vi "loadRecipeOthers.vi"() -> ()   [LabVIEW 2012]
uses:
  <vilib>/Utility/NIReport.llb/NI_report.lvclass
  <vilib>/addons/database/Connection.llb/DB Tools Open Connec (Path).vi
  <vilib>/addons/database/Connection.llb/Conn Execute.vi
  <vilib>/addons/database/Recordset.llb/Rec Destroy - Connection.vi
  <vilib>/Utility/NIReport.llb/Excel/NI_Excel.lvclass
  <vilib>/addons/database/NI_Database_API.lvlib
panel:
  in  "path":path=path "O:/Monitor/Recipe/OTHERS"
  out "filenames":string[](array[string])
  out "appended path":path
  out "data":string[][](array[string])
  out "error out 4":errorcluster
  in  "Cluster":T1
  out "error out 3":errorcluster
  in  "start cell":string="a2"
  out "error out":errorcluster
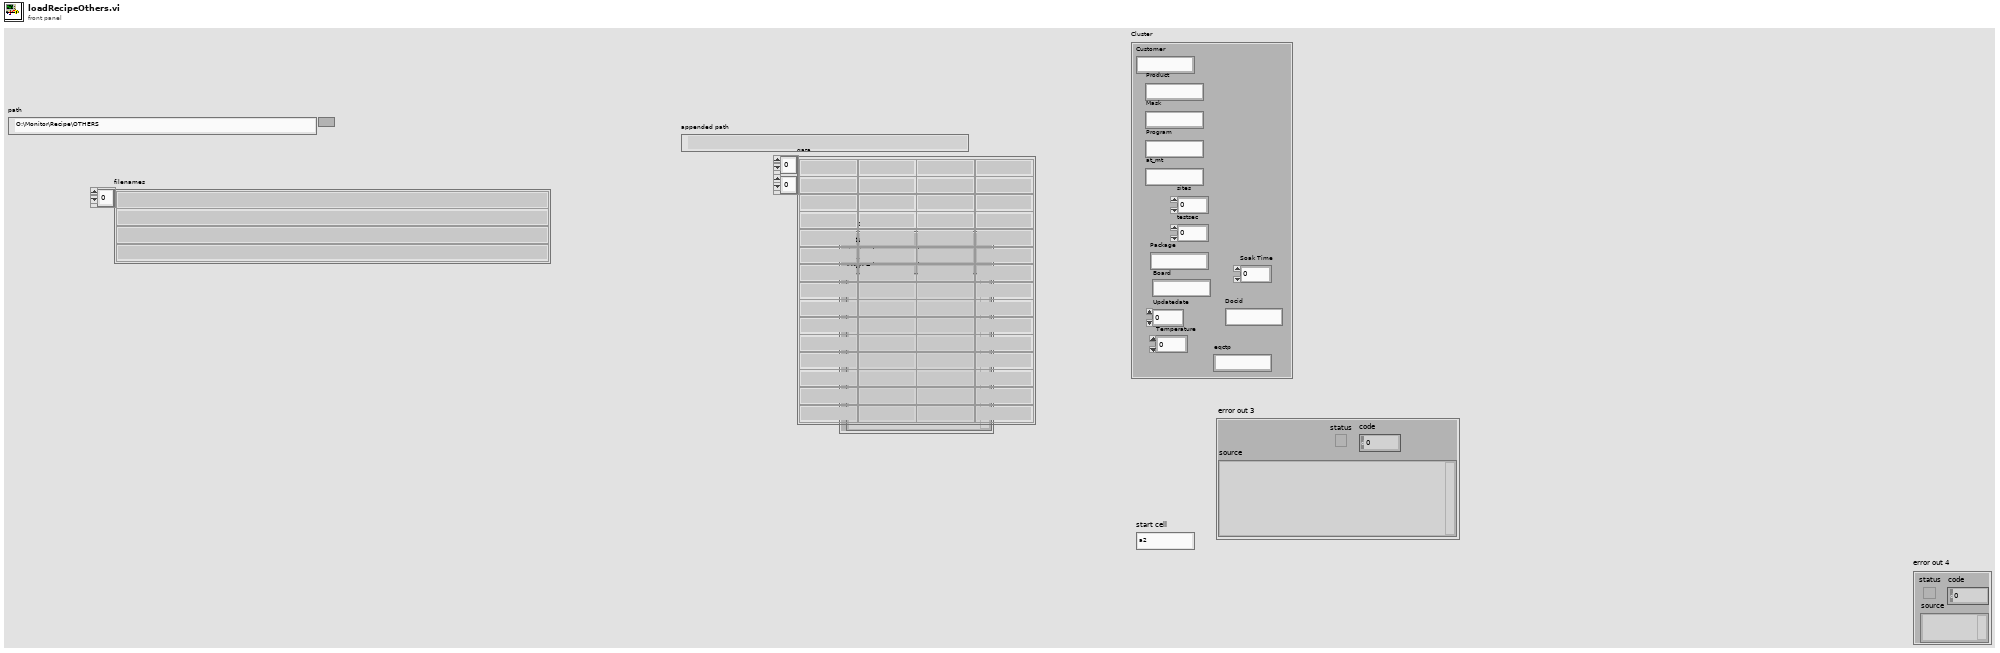
[diagram p1: front panel]
types:
  T1 = cluster{"Customer ":string, "Product":string, "Mask":string, "Program":string, "at_mt":string, "sites ":dbl, "testsec":dbl, "Package":string, "Board ":string, "Updatedate ":dbl, "Temperature":dbl, "Soak Time":dbl, "Docid":string, "eqctp":string}
  T2 = enum16{"Standard Report", "HTML", "Word", "Excel"}
  T3 = typedef "NI_Database_API.lvlib/Conn ObjectReference.ctl" = refnum<k1>
  T4 = typedef "NI_Database_API.lvlib/Rec ObjectReference.ctl" = refnum<k1>
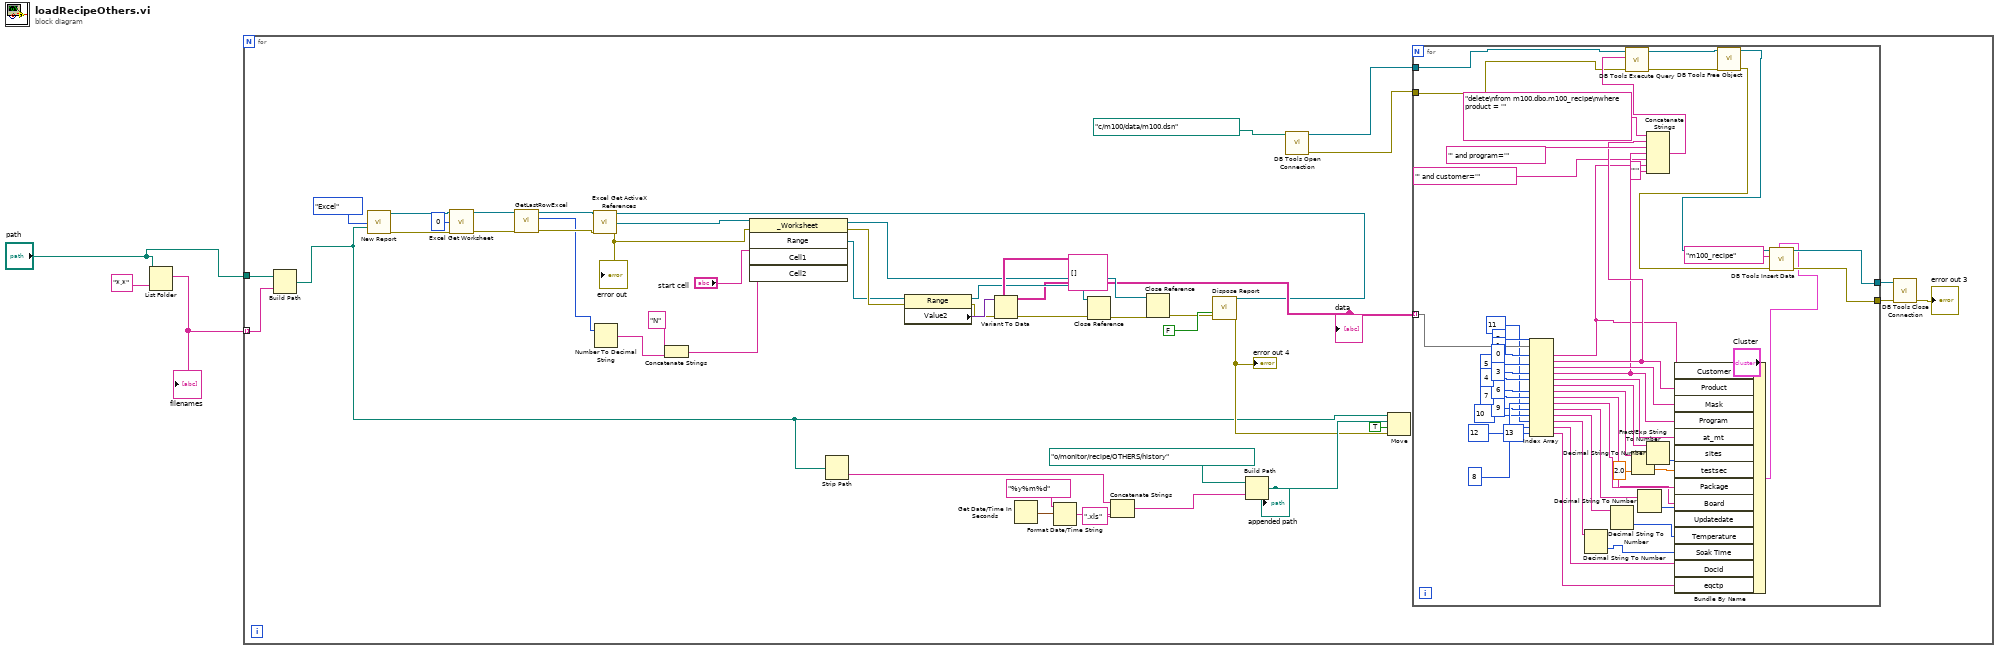
[diagram p0: block diagram]
diagram:
  n1 = List Folder(path="path", pattern="*.*") -> (filenames=w1:string[])  [unwired: 2 in, 3 out]
  "filenames" <- w1
  n2 = for {
    tunnel: "path" -> [w7]
    tunnel: w1 -> [w6] mode=indexing
    n3 = Build Path(base path=w7, name or relative path=w6) -> (appended path=w5:path)
    n4 = call <vilib>:"New Report.vi"("report type"=T2."Excel", "template (empty)"=w5) -> ("report out"=w49:refnum<class "NI_report.lvclass">, "error out"=w48:errorcluster)  [unwired: 12 in]
    n5 = call <vilib>:"Excel Get Worksheet.vi"("report in"=w49, "worksheet index (0)"=0, "error in (no error)"=w48) -> ("report out"=w29:refnum<class "NI_report.lvclass">, "error out"=w28:errorcluster)  [unwired: 11 in]
    n6 = call "GetLastRowExcel.vi"("error in (no error)"=w28, "report in"=w29) -> ("error out"=w26:errorcluster, "row"=w25:i32, "report out"=w27:refnum<class "NI_report.lvclass">)  [unwired: 7 in]
    n7 = call <vilib>:"Excel Get ActiveX References.vi"("report in"=w27, "error in (no error)"=w26) -> ("report out"=w19:refnum<class "NI_report.lvclass">, "Excel._Worksheet"=w45:refnum<k7>, "error out"=w30:errorcluster)  [unwired: 7 in, 4 out]
    "error out" <- w30
    n8 = Number To Decimal String(number=w25) -> (decimal integer string=w23:string)  [unwired: 1 in]
    n9 = Concatenate Strings("N" ("string"), w23) -> (w22:string)
    n10 = invoke class="_Worksheet" method="Range"(reference=w45, error in=w30, "Cell1"="start cell", "Cell2"=w22) -> (reference out=w37:refnum<k7>, error out=w42:errorcluster, "Range"=w41:refnum<k7>)  [unwired: 1 in, 2 out]
    n11 = Strip Path(path=w5) -> (name=w8:string)  [unwired: 1 out]
    n12 = property class="Range"(reference=w41, error in=w42) -> (reference out=w38:refnum<k7>, error out=w43:errorcluster, "Value2"=w44:variant)
    n13 = Variant To Data(error in=w43, type=string[][] [], Variant=w44) -> (data=w31:string[][], error out=w39:errorcluster)
    "data" <- w31
    n14 = Get Date/Time In Seconds() -> (seconds since 1Jan1904=w16:timestamp)
    n15 = Format Date/Time String(time format string (%c)="%y%m%d", seconds (now)=w16) -> (date/time string=w14:string)  [unwired: 1 in]
    n16 = Close Reference(reference=w38, error in (no error)=w39) -> (error out=w36:errorcluster)
    n17 = Concatenate Strings(w8, w14, ".xls" ("string")) -> (w17:string)
    n18 = Close Reference(reference=w37, error in (no error)=w36) -> (error out=w20:errorcluster)
    n19 = call-dynamic "Dispose Report.vi"("report in"=w19, "save changes? (F)"=FALSE, "error in (no error)"=w20) -> ("error out"=w11:errorcluster)  [unwired: 12 in]
    "error out 4" <- w11
    n20 = Build Path(base path=path "o:/monitor/recipe/OTHERS/history", name or relative path=w17) -> (appended path=w12:path)
    "appended path" <- w12
    n21 = call-poly <vilib>:"DB Tools Open Connection.vi"("connection information"=path "c:/m100/data/m100.dsn") -> ("error out"=w9:errorcluster, "connection reference"=w4:T3)  [unwired: 7 in]
    n22 = Move(source path=w5, error in=w11, 9:TRUE ("overwrite (F)"), 10:w12) -> ()  [unwired: 1 in, 3 out]
    n23 = for {
      tunnel: w9 -> [w65]
      tunnel: [w101] -> w33
      tunnel: [w100] -> w32
      tunnel: w31 -> [w99] mode=indexing
      tunnel: w4 -> [w66]
      n24 = Index Array(array=w99, index #1=0 ("index"), index #2=1 ("index"), index #3=2 ("index"), index #4=3 ("index"), index #5=4 ("index"), index #6=5 ("index"), index #7=6 ("index"), index #8=7 ("index"), index #9=8 ("index"), index #10=9 ("index"), index #11=10 ("index"), index #12=11 ("index"), index #13=12 ("index"), index #14=13 ("index")) -> (element #1=w59:string, element #2=w62:string, element #3=w85:string, element #4=w61:string, element #5=w84:string, element #6=w78:string, element #7=w77:string, element #8=w83:string, element #9=w75:string, element #10=w74:string, element #11=w73:string, element #12=w72:string, element #13=w56:string, element #14=w51:string)
      n25 = Decimal String To Number(string=w72) -> (number=w81:i32)  [unwired: 2 in, 1 out]
      n26 = Decimal String To Number(string=w73) -> (number=w80:i32)  [unwired: 2 in, 1 out]
      n27 = Fract/Exp String To Number(string=w77, default (0 dbl)=2.0 ("default (0 DBL)")) -> (number=w76:dbl)  [unwired: 2 in, 1 out]
      n28 = Decimal String To Number(string=w74) -> (number=w79:i32)  [unwired: 2 in, 1 out]
      n29 = Concatenate Strings("delete\nfrom m100.dbo.m100_recipe\nwhere product = '" ("string"), w62, "' and program='" ("string"), w61, "' and customer='" ("string"), w59, "'" ("string")) -> (w67:string)
      n30 = call-poly <vilib>:"DB Tools Execute Query.vi"("error in (no error)"=w65, "SQL query"=w67, "connection reference"=w66) -> ("error out"=w54:errorcluster, "recordset reference"=w55:T4)  [unwired: 5 in]
      n31 = Decimal String To Number(string=w78) -> (number=w71:i32)  [unwired: 2 in, 1 out]
      n32 = Bundle By Name(cluster="Cluster", "Customer"=w59, "Product"=w62, "Mask"=w85, "Program"=w61, "at_mt"=w84, "sites"=w71, "testsec"=w76, "Package"=w83, "Board"=w75, "Updatedate"=w79, "Temperature"=w80, "Soak Time"=w81, "Docid"=w56, "eqctp"=w51) -> (w82:T1)
      n33 = call-poly <vilib>:"DB Tools Free Object.vi"("error in (no error)"=w54, "recordset reference"=w55) -> ("error out"=w63:errorcluster, "connection reference"=w64:T3)  [unwired: 8 in]
      n34 = call <vilib>:"DB Tools Insert Data.vi"("data"=w82, "error in (no error)"=w63, "table"="m100_recipe", "connection reference"=w64) -> ("error out"=w100:errorcluster, "connection reference out"=w101:T3)  [unwired: 6 in]
    }
    n35 = call <vilib>:"DB Tools Close Connection.vi"("error in (no error)"=w32, "connection reference"=w33) -> ("error out"=→"error out 3":errorcluster)  [unwired: 5 in]
  }
